vi "Destroy USR Event SIM.vi"(8 "error in (no error)":errorcluster, 11 "SIMULATED in":refnum<class "SIMULATED.lvclass">) -> (0 "error out":errorcluster, 3 "SIMULATED out":refnum<class "SIMULATED.lvclass">)   [LabVIEW 2019, in "SIMULATED.lvclass"]
uses:
  SIMULATED.lvclass
  SIMULATED.lvclass/SIMULATED.ctl
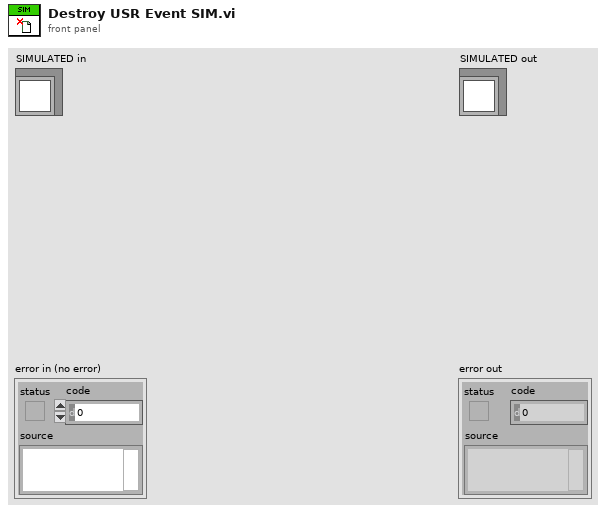
[diagram p1: front panel]
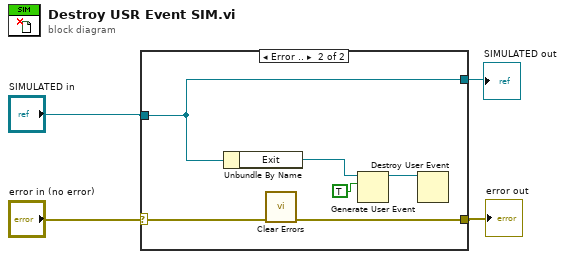
[diagram p0: block diagram]
diagram:
  n1 = case shown="Error .." "error in (no error)" {
    selector: "error in (no error)" -> [w6 w8]
    tunnel: [w6 w7] -> w1
    tunnel: [w5 w12] -> w2
    tunnel: "SIMULATED in" -> [w5 w12]
    frame No Error {
    }
    frame Error {
      n2 = Unbundle By Name(w12) -> ("Exit"=w10:refnum<user-event>)
      n3 = call <vilib>:"Clear Errors.vi"("error in (no error)"=w8) -> ("error out"=w7:errorcluster)  [unwired: 5 in, 1 out]
      n4 = Generate User Event(user event=w10, event data cluster=TRUE ("event data")) -> (user event out=w11:refnum<user-event>)  [unwired: 2 in, 1 out]
      n5 = Destroy User Event(user event=w11) -> ()  [unwired: 1 in, 1 out]
    }
  }
  "error out" <- w1
  "SIMULATED out" <- w2
